vi "Is Terminal on Tunnel.vi"(11 "Terminal in":refnum<vi>) -> (0 "Is Inner Tunnel?":bool, 1 "ClassName of tunnel ref":string, 2 "Terminal is on Tunnel":bool, 3 "Tunnel Ref":refnum<vi>, 4 "Tunnel on Flat Sequence?":bool, 5 "Flat Seq Inner Term":refnum<vi>, 7 "Flat Seq Outer Term":refnum<vi>)   [LabVIEW 2023]
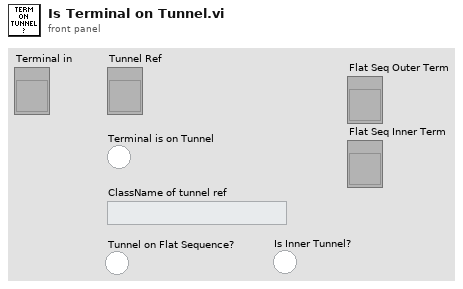
[diagram p1: front panel]
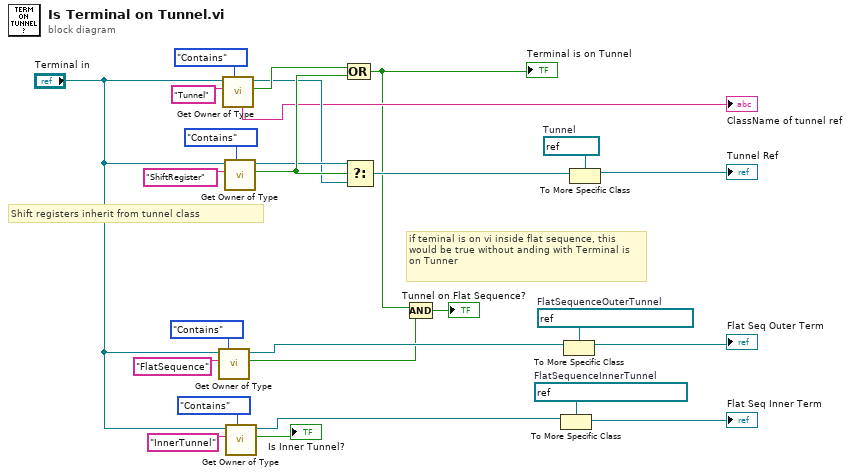
[diagram p0: block diagram]
diagram:
  w10 = refnum<vi> refnum  # FlatSequenceInnerTunnel
  w11 = refnum<vi> refnum  # FlatSequenceOuterTunnel
  w20 = refnum<vi> refnum  # Tunnel
  # "if teminal is on vi inside flat sequence, this would be true without anding with Terminal is on Tunner"
  # "Shift registers inherit from tunnel class"
  n1 = call "Get Owner of Type.vi"("Match Type"=enum16{"Exact Match", "Contains"}."Contains", "Owner Class Name desired"="FlatSequence", "reference"="Terminal in") -> ("Owner of type found?"=w4:bool, "Owner of Type"=w9:refnum<vi>)  [unwired: 4 in, 3 out]
  n2 = call "Get Owner of Type.vi"("Match Type"=enum16{"Exact Match", "Contains"}."Contains", "Owner Class Name desired"="Tunnel", "reference"="Terminal in") -> ("Owner of type found?"=w16:bool, "Owner of Type"=w13:refnum<vi>, "ClassName of ref returned"=→"ClassName of tunnel ref":string)  [unwired: 4 in, 2 out]
  n3 = call "Get Owner of Type.vi"("Match Type"=enum16{"Exact Match", "Contains"}."Contains", "Owner Class Name desired"="ShiftRegister", "reference"="Terminal in") -> ("Owner of type found?"=w15:bool, "Owner of Type"=w14:refnum<vi>)  [unwired: 4 in, 3 out]
  n4 = call "Get Owner of Type.vi"("Match Type"=enum16{"Exact Match", "Contains"}."Contains", "Owner Class Name desired"="InnerTunnel", "reference"="Terminal in") -> ("Owner of type found?"=→"Is Inner Tunnel?":bool, "Owner of Type"=w8:refnum<vi>)  [unwired: 4 in, 3 out]
  n5 = Select(t=w14, s=w15, f=w13) -> (s? t:f=w12:refnum<vi>)
  n6 = Compound Arithmetic op=OR(w16, w15) -> (w1:bool)
  "Terminal is on Tunnel" <- w1
  n7 = Compound Arithmetic op=AND(w1, w4) -> (→"Tunnel on Flat Sequence?":bool)
  n8 = To More Specific Class(target class=w10, reference=w8) -> (specific class reference=→"Flat Seq Inner Term":refnum<vi>)  [unwired: 1 in, 1 out]
  n9 = To More Specific Class(target class=w11, reference=w9) -> (specific class reference=→"Flat Seq Outer Term":refnum<vi>)  [unwired: 1 in, 1 out]
  n10 = To More Specific Class(target class=w20, reference=w12) -> (specific class reference=→"Tunnel Ref":refnum<vi>)  [unwired: 1 in, 1 out]
